vi "PID Turn.vi"(7 "PID gains":T1={"proportional gain (Kc)"=0.008, "integral time (Ti, min)"=0.0, "derivative time (Td, min)"=0.0013}, 8 "F gain":dbl=0.5, 9 "Reset gyro":bool, 10 "Error Tolerance +/- (3)":dbl=2.5, 11 "Setpoint":dbl) -> (0 "Done":bool, 2 "Output":dbl, 3 "Angel out":dbl)   [LabVIEW 2015]
uses:
  <vilib>/addons/control/pid/pid.llb/PID Structure Conversion (DBL).vi
  <vilib>/Rock Robotics/WPI/Utilities/WPI_GetSetVariantRefNum.vi
  <vilib>/addons/control/pid/pid.llb/PID Control Input Filter (DBL).vi
  <vilib>/addons/control/pid/pid.llb/PID (DBL).vi
  <vilib>/addons/control/pid/NI_PID_pid.lvlib
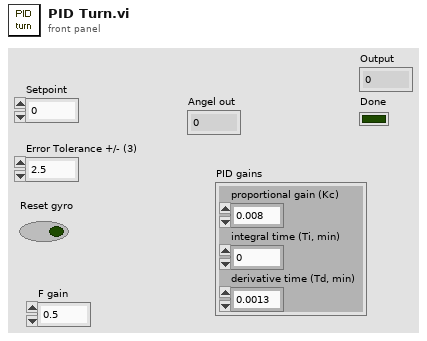
[diagram p1: front panel]
types:
  T1 = cluster{"proportional gain (Kc)":dbl, "integral time (Ti, min)":dbl, "derivative time (Td, min)":dbl}
  T2 = typedef "WPI_GyroDevRef.ctl" = cluster{"DevStatus":errorcluster, "Analog Channel":T3, "Offset":dbl, "Gain (VoltsPerDegree/Second)":dbl, "Gyro Type":enum16{"Analog", "XRS450"}, "Handle":i32, "SPI Bus":T4, "Device Found":bool, "Sample Rate":dbl, "Calibrate On Open":bool}
  T3 = typedef "FPGA_AIChannel.ctl" = enum8{"AI 0", "AI 1", "AI 2", "AI 3", "AI MXP 0", "AI MXP 1", "AI MXP 2", "AI MXP 3", "Invalid"}
  T4 = typedef "spi_bus.ctl" = enum16{"SPI On-Board, CS0", "SPI On-Board, CS1", "SPI On-Board, CS2", "SPI On-Board, CS3", "SPI MXP", "Invalid"}
  T5 = typedef "WPI_RobotDriveDevRef.ctl" = cluster{"DevStatus":errorcluster, "Motors[]":T6[], "Square Inputs":bool, "Max Output":dbl}
  T6 = typedef "WPI_MotorControlDeviceRef.ctl" = cluster{"DeviceStatus":errorcluster, "Type":T7, "PWM":cluster{"PWM Channel":T8, "DeadBand":T9}, "CAN":cluster{"Device Number":u8, "Control Mode":T10, "Semaphore":T11, "Max Vout":dbl, "TalonSRX Control Mode":T12}, "Invert":bool}
  T7 = typedef "WPI_MotorControlType.ctl" = enum16{"PWM", "CAN", "CANTalonSRX"}
  T8 = typedef "FPGA_DIOPWMChannel.ctl" = enum8{"PWM 0", "PWM 1", "PWM 2", "PWM 3", "PWM 4", "PWM 5", "PWM 6", "PWM 7", "PWM 8", "PWM 9", "PWM MXP 0", "PWM MXP 1", "PWM MXP 2", "PWM MXP 3", "PWM MXP 4", "PWM MXP 5", "PWM MXP 6", "PWM MXP 7", "PWM MXP 8", "PWM MXP 9", "Invalid"}
  T9 = typedef "WPI_PWMDeadband.ctl" = cluster{"Name":string, "maxPositivePwm":i32, "minPositivePwm":i32, "centerPwm":i32, "maxNegativePwm":i32, "minNegativePwm":i32, "angularRange":u16}
  T10 = typedef "WPI_CANJaguar_ControlMode.ctl" = enum8{"Percent VBus", "Current", "Speed", "Position", "Voltage"}
  T11 = typedef "Semaphore RefNum" = refnum<k1>
  T12 = typedef "WPI_CANTalonSRX_APIControlMode.ctl" = enum8{"Percent VBus", "Speed", "Position", "Slave", "Unchanged / Invalid", "Voltage Compensation", "Current", "Motion Profile"}
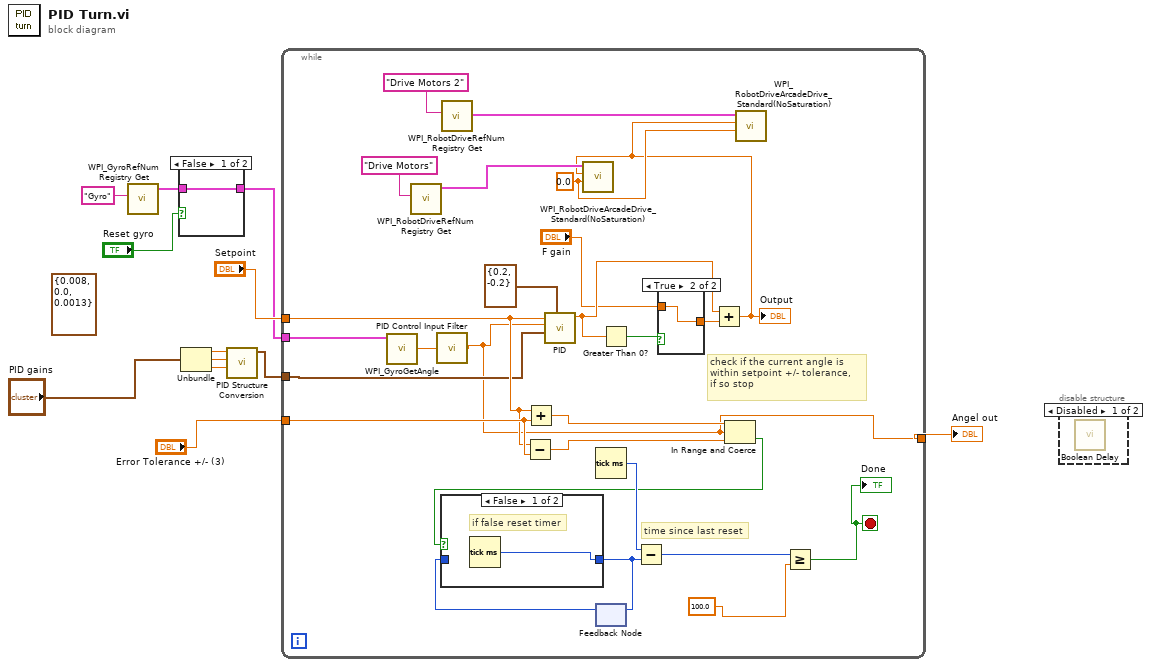
[diagram p0: block diagram]
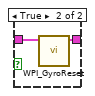
[diagram p3: hidden frame]
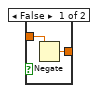
[diagram p5: hidden frame]
diagram:
  (unwired) T1 {"proportional gain (Kc)"=0.008, "integral time (Ti, min)"=0.0, "derivative time (Td, min)"=0.0013} ("PID gains")
  n1 = call <vilib>:"WPI_GyroRefNum Registry Get.vi"("refnum name"="Gyro") -> ("GyroDevRef"=w5:T2)  [unwired: 9 in, 1 out]
  n2 = case shown="False" "Reset gyro" {
    tunnel: w5 -> [w13 w15]
    tunnel: [w13 w14] -> w4
    frame False {
    }
    frame True {
      n3 = call <vilib>:"WPI_GyroReset.vi"("GyroDevRef"=w15) -> ("GyroDevRef"=w14:T2)  [unwired: 9 in, 1 out]
    }
  }
  n4 = Unbundle("PID gains") -> ("proportional gain (Kc)"=w10:dbl, "integral time (Ti, min)"=w11:dbl, "derivative time (Td, min)"=w12:dbl)
  n5 = call-poly <vilib>:"PID Structure Conversion.vi"("derivative"=w12, "integral"=w11, "proportional"=w10) -> ("PID gains"=w8:T1)  [unwired: 8 in]
  n6 = while {
    tunnel: "Setpoint" -> [w37]
    tunnel: w8 -> [w36]
    tunnel: "Error Tolerance +/- (3)" -> [w38]
    tunnel: w4 -> [w31]
    tunnel: [w30] -> w2
    stop <- w16 stop-if-true
    w27 = 0.0 ("Y axis value")
    # "time since last reset"
    # "check if the current angle is\nwithin setpoint +/- tolerance,\nif so stop"
    n7 = call <vilib>:"WPI_GyroGetAngle.vi"("GyroDevRef"=w31) -> ("Angle"=w32:dbl)  [unwired: 6 in, 4 out]
    n8 = call <vilib>:"WPI_RobotDriveRefNum Registry Get.vi"("refnum name"="Drive Motors") -> ("RobotDriveDevRef"=w28:T5)  [unwired: 1 in, 9 out]
    n9 = call-poly <vilib>:"PID Control Input Filter.vi"("input"=w32) -> ("output"=w30:dbl)  [unwired: 4 in]
    n10 = call <vilib>:"WPI_RobotDriveRefNum Registry Get.vi"("refnum name"="Drive Motors 2") -> ("RobotDriveDevRef"=w29:T5)  [unwired: 1 in, 9 out]
    n11 = Subtract(x=w37, y=w38) -> (x-y=w39:dbl)
    n12 = Add(x=w37, y=w38) -> (x+y=w40:dbl)
    n13 = call-poly <vilib>:"PID.vi"("output range"=cluster{"output high":dbl, "output low":dbl} {"output high"=0.2, "output low"=-0.2}, "PID gains"=w36, "process variable"=w30, "setpoint"=w37) -> ("output"=w34:dbl)  [unwired: 6 in, 1 out]
    n14 = Tick Count (ms)() -> (millisecond timer value=w18:u32)
    n15 = feedback #1() -> (w19:u32)  [unwired: 1 in]
    n16 = Greater Than 0?(x=w34) -> (x > 0?=w35:bool)
    n17 = case shown="True" w35 {
      tunnel: [w44 w46] -> w33
      tunnel: "F gain" -> [w45 w46]
      frame False {
        n18 = Negate(x=w45) -> (-x=w44:dbl)
      }
      frame True {
      }
    }
    n19 = Add(x=w34, y=w33) -> (x+y=w26:dbl)
    "Output" <- w26
    n20 = call <vilib>:"WPI_RobotDriveArcadeDrive_Standard(NoSaturation).vi"("Y axis value"=w27, "X axis value"=w26, "RobotDriveDevRef"=w28) -> ()  [unwired: 1 in, 8 out]
    n21 = In Range and Coerce(upper limit=w40, x=w30, lower limit=w39) -> (In Range?=w17:bool)  [unwired: 1 out]
    n22 = case shown="False" w17 {
      tunnel: [w42 w43] -> w20
      tunnel: w19 -> [_ w43]
      frame False {
        # "if false reset timer"
        n23 = Tick Count (ms)() -> (millisecond timer value=w42:u32)
      }
      frame True {
        # "if true don't reset timer"
      }
    }
    n24 = feedback-in #1(w20) -> ()
    n25 = Subtract(x=w18, y=w20) -> (x-y=w21:u32)
    n26 = call <vilib>:"WPI_RobotDriveArcadeDrive_Standard(NoSaturation).vi"("Y axis value"=w27, "X axis value"=w26, "RobotDriveDevRef"=w29) -> ()  [unwired: 1 in, 8 out]
    n27 = Greater Or Equal?(x=w21, y=100.0 ("Delay (ms)")) -> (x >= y?=w16:bool)
    "Done" <- w16
  }
  "Angel out" <- w2
  n28 = disable-structure shown="Disabled" {
    frame Disabled {
      n29 = call "Boolean Delay.vi"() -> ()  [unwired: 3 in, 1 out]
    }
    frame Enabled {
    }
  }
